vi "Initialization.vi"(5 "Communication Port":i32(ring) items=["COM1", "USB"], 11 "error in":errorcluster, 13 "System Message Refnum":refnum<vi>) -> (4 "VISA OUT":refnum<visa-resource-name>, 6 "Communication Port Out":i32(ring) items=["COM1", "USB"], 15 "error out":errorcluster)   [LabVIEW 2018, in "Stage Controller.lvlib"]
doc: "VI initializes and configues the MAC5000; the user chooses whether communication with the MAC5000 occurs over the Serial Port(RS232) or the USB port. This VI should be run once at the beginning of a larger program.\n\nNote: \nSerial Port communication occurs over Serial Port 1; if the user wants to use a different Serial Port the VISA Resource name needs to be changed in the block diagram from ASRL1::INSTR to ASRL#::INSTR where # is the number of the Serial Port.\nTo use USB communication, the user needs to set up the VISA protocol using the VISA driver development wizard. After setting up the VISA driver, the user needs to enter the correct VISA resource name in the block diagram. Note the VISA resource name is specific to a particular USB Bus; if the MAC5000 is plugged into another USB bus the user needs to set up the VISA resource name again."
uses:
  <vilib>/Instr/_visa.llb/VISA Configure Serial Port (Instr).vi
  Stage Controller.lvlib
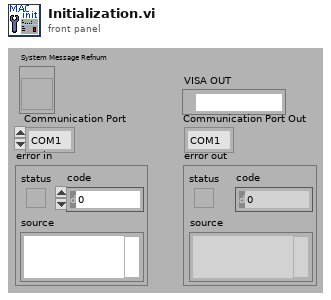
[diagram p1: front panel]
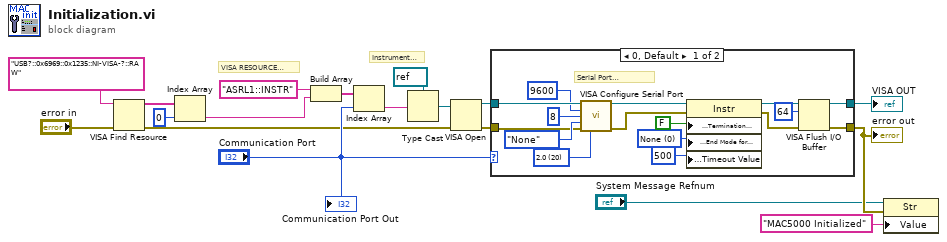
[diagram p0: block diagram]
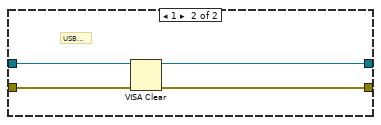
[diagram p2: hidden frame]
diagram:
  # "Instrument Class"
  # "VISA RESOURCE NAMES"
  n1 = VISA Find Resource(8:"error in", 11:"USB?::0x6969::0x1235::NI-VISA-?::RAW") -> (0:w8:errorcluster, 3:w6:string[])  [unwired: 1 in, 1 out]
  n2 = Index Array(array=w6, index=0) -> (element=w5:string)
  n3 = Build Array("ASRL1::INSTR", w5) -> (w16:string[])
  n4 = Index Array(array=w16, index="Communication Port") -> (element=w15:string)
  n5 = Type Cast(type=refnum<visa-resource-name> refnum, x=w15) -> (*(type *) &x=w14:refnum<visa-resource-name>)
  n6 = VISA Open(error in (no error)=w8, VISA resource name=w14) -> (VISA resource name=w12:refnum<visa-resource-name>, error out=w11:errorcluster)  [unwired: 3 in]
  n7 = case shown="0, Default" "Communication Port" {
    tunnel: w11 -> [w30 w37]
    tunnel: w12 -> [w34 w38]
    tunnel: [w21 w36] -> w3
    tunnel: [w20 w35] -> w10
    frame 0, Default {
      w19 = u16 20 items=["1.0"=10, "1.5"=15, "2.0"=20] ("stop bits (10: 1 bit)")
      w28 = u16 0 items=["None", "LastBit", "TermChar"] ("Serial Settings:Serial End Mode for Reads")
      # "Serial Port Configuration"
      n8 = call-poly "VISA Configure Serial Port"("VISA resource name"=w34, "baud rate (9600)"=u32 9600, "data bits (8)"=u16 8, "parity (0:none)"=enum16{"None", "Odd", "Even", "Mark", "Space"}."None", "error in (no error)"=w30, "stop bits (10: 1 bit)"=w19) -> ("VISA resource name out"=w26:refnum<visa-resource-name>, "error out"=w25:errorcluster)  [unwired: 8 in]
      n9 = property class="Instr"(reference=w26, error in=w25, "Message Based Settings:Termination Character Enable"=FALSE, "Serial Settings:End Mode for Reads"=w28, "General Settings:Timeout Value"=u32 500) -> (reference out=w23:refnum<visa-resource-name>, error out=w22:errorcluster)
      n10 = VISA Flush I/O Buffer(VISA resource name=w23, mask (16)=u16 64, error in (no error)=w22) -> (VISA resource name out=w20:refnum<visa-resource-name>, error out=w21:errorcluster)
    }
    frame 1 {
      # "USB Port"
      n11 = VISA Clear(VISA resource name=w38, error in (no error)=w37) -> (VISA resource name out=w35:refnum<visa-resource-name>, error out=w36:errorcluster)
    }
  }
  "error out" <- w3
  "VISA OUT" <- w10
  n12 = property class="Str"(reference="System Message Refnum", error in=w3, "Value"="MAC5000 Initialized") -> ()  [unwired: 2 out]
  "Communication Port Out" <- "Communication Port"
